vi "FWHM-Testes.vi"() -> ()   [LabVIEW 2014]
uses:
  <vilib>/Analysis/NI_AALPro.lvlib
panel:
  out "best fit":dynamicdata(graph)
  out "standard deviation":dbl
  out "center":dbl
  out "amplitude":dbl
  out "XY Graph":cluster{"X Values":dbl[], "Y Values":dbl[]}(graph)
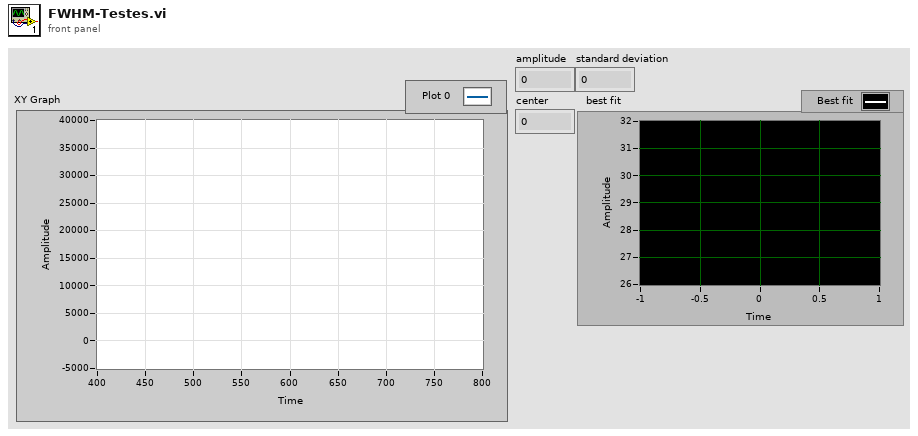
[diagram p1: front panel]
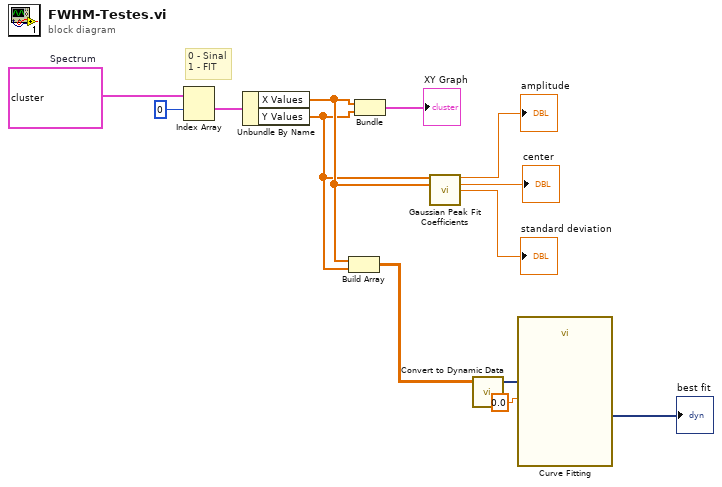
[diagram p0: block diagram]
diagram:
  w13 = cluster{"X Values":dbl[], "Y Values":dbl[]}[] [{"X Values"=array[1165 elements], "Y Values"=array[1165 elements]}, {"X Values"=array[1000 elements], "Y Values"=array[1000 elements]}]  # Spectrum
  # "0 - Sinal\n1 - FIT"
  n1 = Index Array(array=w13, index #1=0 ("index")) -> (element #1=w11:cluster{"X Values":dbl[], "Y Values":dbl[]})  [unwired: 1 in, 1 out]
  n2 = Unbundle By Name(w11) -> ("X Values"=w6:dbl[], "Y Values"=w5:dbl[])
  n3 = Build Array(w6, w5) -> (w4:dbl[][])
  n4 = Bundle("X Values"=w6, "Y Values"=w5) -> (→"XY Graph":cluster{"X Values":dbl[], "Y Values":dbl[]})  [unwired: 1 in]
  n5 = call <vilib>:"Gaussian Peak Fit Coefficients.vi"("Y"=w5, "X"=w6) -> ("amplitude"=→"amplitude":dbl, "center"=→"center":dbl, "standard deviation"=→"standard deviation":dbl)  [unwired: 10 in, 1 out]
  n6 = call "Convert to Dynamic Data"("2D Array"=w4) -> ("Dynamic Data Type"=w3:dynamicdata)  [unwired: 3 in]
  n7 = call "Curve Fitting"("Locations"=0.0, "Signals"=w3) -> ("best fit"=→"best fit":dynamicdata)  [unwired: 6 in, 3 out]
